vi "GetTests.vi"(8 "error in (no error)":errorcluster, 11 "TestSuite in":refnum<class "TestSuite.lvclass">) -> (0 "error out":errorcluster, 2 "tests":refnum<class>[](array[class]), 3 "TestSuite in":refnum<class "TestSuite.lvclass">)   [LabVIEW 2013, in "TestSuite.lvclass"]
doc: "Gets the test members of testSuite. 'tests' can be testCase or testSuite objects (can be mixed)."
uses:
  TestSuite.lvclass
  TestSuite.lvclass/TestSuite.ctl
panel:
  # "JKI VI Tester for LabVIEW\nhttp://jkisoft.com/vi-tester\nCopyright (C) 2007-2009, JKI <info@jkisoft.com>\nALL RIGHTS RESERVED"
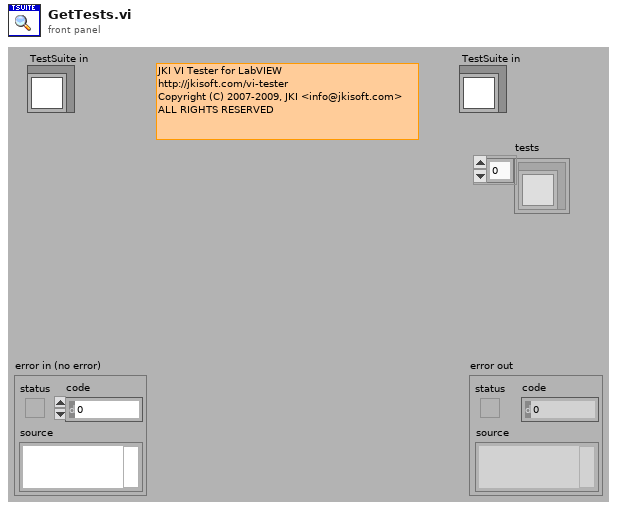
[diagram p1: front panel]
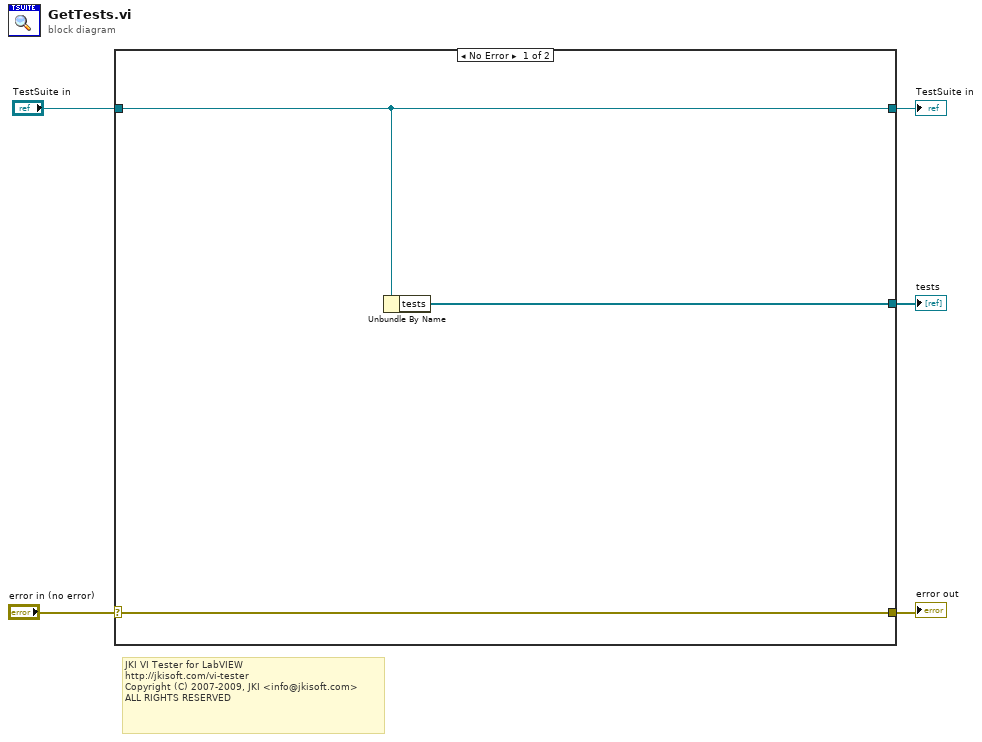
[diagram p0: block diagram]
diagram:
  # "JKI VI Tester for LabVIEW\nhttp://jkisoft.com/vi-tester\nCopyright (C) 2007-2009, JKI <info@jkisoft.com>\nALL RIGHTS RESERVED"
  n1 = case shown="No Error" "error in (no error)" {
    selector: "error in (no error)" -> [w7 w10]
    tunnel: [w7 w10] -> w4
    tunnel: [w6 w9] -> w2
    tunnel: "TestSuite in" -> [w6 w9]
    tunnel: [w8 _] -> w1
    frame No Error {
      n2 = Unbundle By Name(w6) -> ("tests"=w8:refnum<class>[])
    }
    frame Error {
    }
  }
  "error out" <- w4
  "TestSuite in" <- w2
  "tests" <- w1
